vi "Test_Cmd_1.vi"(8 "error in":errorcluster, 10 "Write":T2={"Write"="", "Fbk?"=TRUE}, 11 "Port":string="COM13") -> (0 "error out":errorcluster, 2 "Read":T1)   [LabVIEW 2016, in "Serial_G.lvlib"]
doc: "Tests a cmd"
uses:
  Serial_G.lvlib
  Controls/Cmd_Tx.ctl
  Controls/Cmd_Rx.ctl
  Controls/PortConfig.ctl
panel:
  in  "Log?":bool
  out "Port?":bool
  # "Serial Communication Driver - Cmd (Tx-Rx)"
  # "Cmd                                                                   w/Read?"
  # "Response                                                            Exec time   Timeout?"
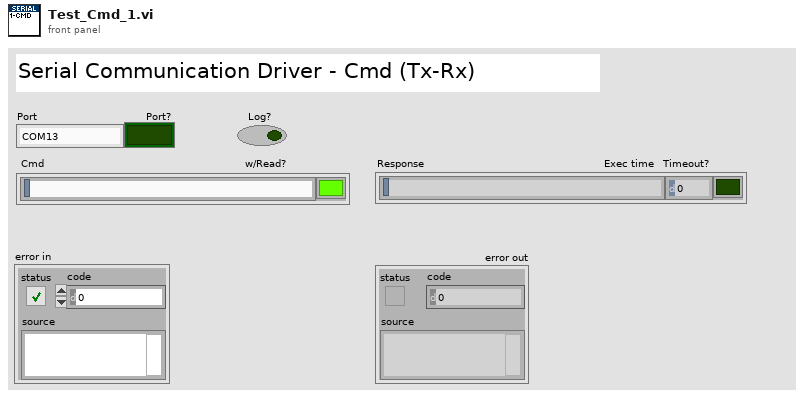
[diagram p1: front panel]
types:
  T1 = typedef "Serial_G.lvlib/Cmd_Rx.ctl" = cluster{"Read":string, "ExecTime (ms)":i32, "Timeout?":bool}
  T2 = typedef "Serial_G.lvlib/Cmd_Tx.ctl" = cluster{"Write":string, "Fbk?":bool}
  T3 = typedef "Serial_G.lvlib/PortConfig.ctl" = cluster{"Baud rate":u32, "Parity":enum16{"None", "Odd", "Even", "Mark", "Space"}, "Data bits":u16, "Stop bits":u16, "Flow control":u16}
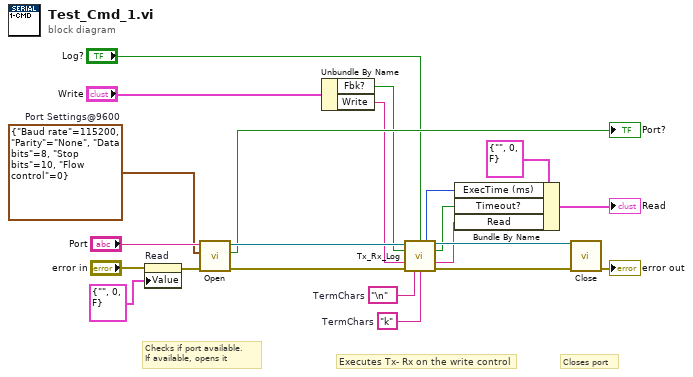
[diagram p0: block diagram]
diagram:
  w1 = "k"  # TermChars
  w3 = T3 {"Baud rate"=115200, "Parity"=enum."None", "Data bits"=8, "Stop bits"=10, "Flow control"=0}  # Port Settings@9600
  w17 = "\n"  # TermChars
  # "Closes port"
  # "Executes Tx- Rx on the write control"
  # "Checks if port available.\nIf available, opens it"
  n1 = property on="Read" class="Clust (strict)"(error in="error in", "Value"=T1 {"Read"="", "ExecTime (ms)"=0, "Timeout?"=FALSE} ("Read")) -> (error out=w14:errorcluster)  [unwired: 1 in, 1 out]
  n2 = call "Open.vi"("error in"=w14, "ConfigPort (9600,0,8,1)"=w3, "Port(Alias)"="Port") -> ("error out"=w22:errorcluster, "PortFound?"=→"Port?":bool, "VISA out"=w21:refnum<visa-resource-name>)  [unwired: 5 in, 1 out]
  n3 = Unbundle By Name("Write") -> ("Fbk?"=w10:bool, "Write"=w9:string)
  n4 = call "Tx_Rx_Log.vi"("VISA in"=w21, "Log?"="Log?", "Fbk? (T)"=w10, "Write"=w9, "error in"=w22, "TermChar (\\n)"=w17, "Wait for? (\\n)"=w1) -> ("ExecTime(ms)"=w4:i32, "VISA out"=w20:refnum<visa-resource-name>, "Timeout?"=w5:bool, "Read"=w6:string, "error out"=w18:errorcluster)  [unwired: 4 in]
  n5 = Bundle By Name(cluster=T1 {"Read"="", "ExecTime (ms)"=0, "Timeout?"=FALSE} ("Read"), "ExecTime (ms)"=w4, "Timeout?"=w5, "Read"=w6) -> (→"Read":T1)
  n6 = call "Close.vi"("error in"=w18, "VISA in"=w20) -> ("error out"=→"error out":errorcluster)  [unwired: 9 in]
